vi "Measure Immediate.vi"(8 "error in":errorcluster, 9 "Source":i32(ring) items=["Input Channel 1", "Input Channel 2", "Input Channel 3", "Input Channel 4", "Calc Channel 1", "Calc Channel 2", "Calc Channel 3", "Calc Channel 4", "Ref Channel 1", "Ref Channel 2", "Ref Channel 3", "Ref Channel 4"], 10 "Measurement":i32(ring) items=["AC RMS", "Amplitude", "Average", "Cycle Average", "Cycle Frequency", "Cycle Period", "Cycle RMS", "DC RMS", "Estimated Number of Bits", "Falling Edges", "Fall Overshoot", "Fall Preshoot", "Frequency", "Fall Crossing Time", "Fall Time", "High", "Low", "Maximum", "Minimum", "Mid", "Negative Duty", "Negative Width", "Positive Duty", "Period", "Phase", "Peak to Peak", "Positive Width", "Rising Edges", "Rise Overshoot", "Rise Preshoot", "Rise Crossing Time", "Rise Time", "Standard Deviation", "Spurious Free Dynamic Range", "Signal to Noise+Distortion", "Signal to Noise", "Total Harmonic Distortion", "Time of Maximum", "Time of Minimum"], 11 "Instrument Handle In":i32) -> (0 "error out":errorcluster, 2 "Result":dbl, 3 "Instrument Handle Out":i32)   [LabVIEW 8.6, in "ZTScopeM.lvlib"]
doc: "Perform a measurement and read the result."
uses:
  ZTScopeM.lvlib
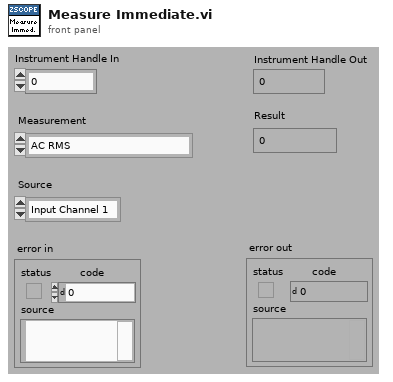
[diagram p1: front panel]
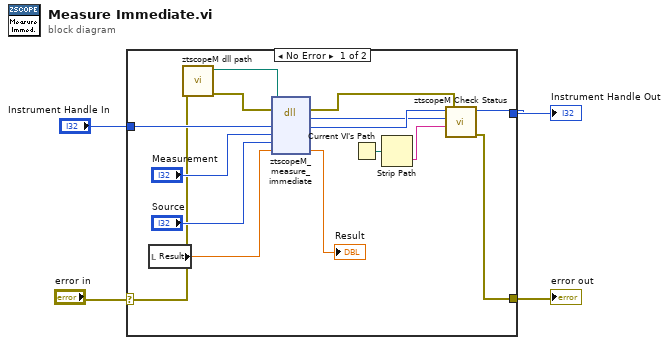
[diagram p0: block diagram]
diagram:
  n1 = case shown="No Error" "error in" {
    selector: "error in" -> [w8 w21]
    tunnel: [w10 w21] -> w1
    tunnel: "Instrument Handle In" -> [w19 w20]
    tunnel: [w9 w20] -> w3
    frame #0 {
      n2 = local read "Result"() -> (w16:dbl)
      n3 = call "ztscopeM dll path.vi"("error in (no error)"=w8) -> ("error out"=w6:errorcluster, "<instrument>.dll path"=w7:path)  [unwired: 9 in]
      n4 = dll-call lib="C:/Program Files (x86)/National Instruments/LabVIEW 2013/instr.lib/ztscopem/ztscopeM.dll" fn="ztscopeM_measure_immediate"(path in=w7, error in=w6, "instrumentHandle"=w19, "Measurement"="Measurement", "source"="Source", "result"=w16) -> (error out=w5:errorcluster, w11:i32, "instrumentHandle"=w12:i32, "result"=→"Result":dbl)  [unwired: 3 in, 1 out]
      n5 = Current VI's Path() -> (path=w14:path)
      n6 = Strip Path(path=w14) -> (name=w13:string)  [unwired: 1 out]
      n7 = call "ztscopeM Check Status.vi"("error in"=w5, "name of VI"=w13, "status (return code)"=w11, "instrument handle in"=w12) -> ("error out"=w10:errorcluster, "instrument handle out"=w9:i32)  [unwired: 2 in]
    }
    frame #1 {
    }
  }
  "Instrument Handle Out" <- w3
  "error out" <- w1
